vi "Edge Detect.vi"(4 "init":bool, 6 "Type":enum16{"0->1", "1->0"}(ring), 11 "Data In":i32) -> (3 "Found":bool)   [LabVIEW 2017]
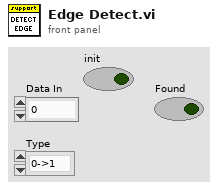
[diagram p1: front panel]
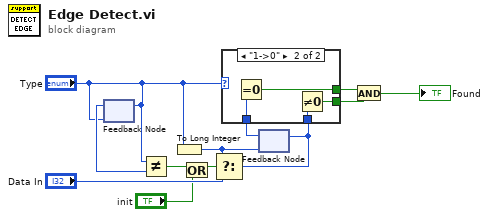
[diagram p0: block diagram]
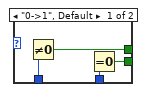
[diagram p2: hidden frame]
diagram:
  n1 = feedback-in #1("Type") -> ()
  n2 = feedback #1("Type") -> (w5:enum16{"0->1", "1->0"})
  n3 = Not Equal?(x="Type", y=w5) -> (x != y?=w6:bool)
  n4 = To Long Integer(number="Type") -> (32bit integer=w3:i32)
  n5 = Or(x=w6, y="init") -> (x .or. y?=w2:bool)
  n6 = Select(t=w3, s=w2, f="Data In") -> (s? t:f=w7:i32)
  n7 = feedback #2(w3) -> (w9:i32)
  n8 = case shown="\"1->0\"" "Type" {
    tunnel: [w16 w20] -> w11
    tunnel: [w15 w19] -> w10
    tunnel: w7 -> [w14 w18]
    tunnel: w9 -> [w13 w17]
    frame "0->1", Default {
      n9 = Not Equal To 0?(x=w13) -> (x != 0?=w16:bool)
      n10 = Equal To 0?(x=w14) -> (x = 0?=w15:bool)
    }
    frame "1->0" {
      n11 = Equal To 0?(x=w17) -> (x = 0?=w20:bool)
      n12 = Not Equal To 0?(x=w18) -> (x != 0?=w19:bool)
    }
  }
  n13 = feedback-in #2(w7) -> ()
  n14 = And(x=w11, y=w10) -> (x .and. y?=→"Found":bool)
